vi "Control Loop.vi"(8 "error in (no error)":errorcluster, 11 "FormulaG App in":refnum<class "FormulaG App.lvclass">) -> (0 "error out":errorcluster)   [LabVIEW 2020, in "FormulaG.lvlib" / "FormulaG App.lvclass"]
uses:
  FormulaG App.lvclass
  FormulaG App.lvclass/FormulaG App.ctl
  State Update.ctl
  FormulaG-Common/Car State.ctl
  FormulaG-Common/Ranges.ctl
  FormulaG-Common/Car Info.ctl
  FormulaG-Common/Car Control.ctl
  FormulaG API/FormulaG API.lvclass
  FormulaG-Common/FormulaG-Common.lvlib
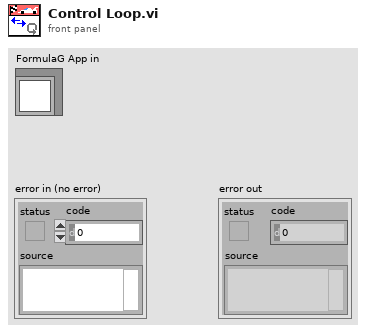
[diagram p1: front panel]
types:
  T1 = typedef "FormulaG-Common.lvlib/Control VI.ctl" = refnum<vi>
  T2 = typedef "FormulaG.lvlib/FormulaG App.lvclass/State Update.ctl" = cluster{"Car State":T3, "Car Control":T6, "Update Rate":dbl, "error":errorcluster}
  T3 = typedef "FormulaG-Common.lvlib/Car State.ctl" = cluster{"Ranges":T4, "Car Info":T5, "Current Lap":dbl, "Last Lap":dbl, "Lap":u8}
  T4 = typedef "FormulaG-Common.lvlib/Ranges.ctl" = cluster{"Front":sgl[], "Rear":sgl[]}
  T5 = typedef "FormulaG-Common.lvlib/Car Info.ctl" = cluster{"Speed":sgl, "X":sgl, "Y":sgl, "Heading":sgl}
  T6 = typedef "FormulaG-Common.lvlib/Car Control.ctl" = cluster{"Steering (-1 to 1)":sgl, "Throttle (0 to 1)":sgl}
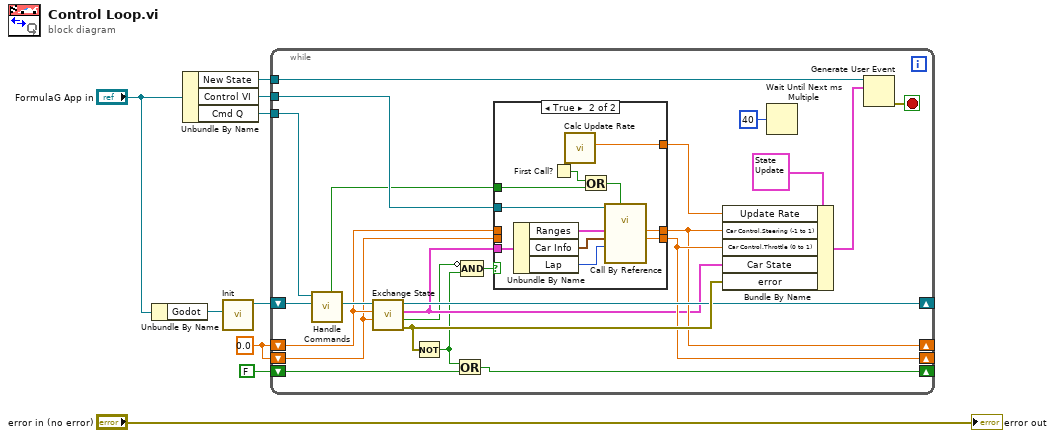
[diagram p0: block diagram]
diagram:
  w3 = sgl 0.0 ("Throttle (0 to 1)")
  n1 = Unbundle By Name("FormulaG App in") -> ("Godot"=w8:refnum<class "GodotServer.lvclass">)
  n2 = Unbundle By Name("FormulaG App in") -> ("New State"=w5:refnum<user-event>, "Control VI"=w6:T1, "Cmd Q"=w4:refnum<queue>)
  n3 = call "Init.vi"("Godot"=w8) -> ("FormulaG API out"=w2:refnum<class "FormulaG API.lvclass">)  [unwired: 9 in, 1 out]
  n4 = while {
    shift-right: [w28] -> _
    shift-left: w2 -> [w30]
    tunnel: w6 -> [w29]
    tunnel: w5 -> [w27]
    tunnel: w4 -> [w22]
    shift-right: [w20] -> _
    shift-left: w3 -> [w14]
    shift-right: [w19] -> _
    shift-left: w3 -> [w15]
    shift-right: [w16] -> _
    shift-left: FALSE -> [w18]
    stop <- w25 stop-if-true
    n5 = call "Handle Commands.vi"("FormulaG API in"=w30, "Cmd Q"=w22) -> ("FormulaG API"=w23:refnum<class "FormulaG API.lvclass">, "Reset"=w21:bool)  [unwired: 8 in]
    n6 = call "Exchange State.vi"("Throttle"=w14, "Steering"=w15, "FormulaG API in"=w23) -> ("error out"=w32:errorcluster, "Paused"=w10:bool, "Car State"=w17:T3, "FormulaG API out"=w28:refnum<class "FormulaG API.lvclass">)  [unwired: 5 in]
    n7 = Not(x=w32) -> (.not. x?=w12:bool)
    n8 = Or(x=w12, y=w18) -> (x .or. y?=w16:bool)
    n9 = Compound Arithmetic op=AND(invert w10, w12) -> (w11:bool)
    n10 = case shown="True" w11 {
      tunnel: w29 -> [_ w45]
      tunnel: w21 -> [_ w40]
      tunnel: [w33 w38] -> w20
      tunnel: [w34 w37] -> w19
      tunnel: w17 -> [_ w36]
      tunnel: w15 -> [w34 _]
      tunnel: w14 -> [w33 _]
      tunnel: [_ w35] -> w13
      frame False {
      }
      frame True {
        n11 = Unbundle By Name(w36) -> ("Ranges"=w44:T4, "Car Info"=w43:T5, "Lap"=w39:u8)
        n12 = First Call?() -> (First Call?: T/F=w42:bool)
        n13 = call "Calc Update Rate.vi"() -> ("Update Rate"=w35:dbl)  [unwired: 11 in]
        n14 = Or(x=w42, y=w40) -> (x .or. y?=w41:bool)
        n15 = call-by-ref "?"(reference=w45, "Reset"=w41, "Lap"=w39, "Car Info"=w43, "Ranges"=w44) -> ("Throttle (0 to 1)"=w38:sgl, "Steering (-1 to 1)"=w37:sgl)  [unwired: 7 in, 2 out]
      }
    }
    n16 = Bundle By Name(cluster=T2 {"Car State"={"Ranges"={"Front"=[], "Rear"=[]}, "Car Info"={"Speed"=0.0, "X"=0.0, "Y"=0.0, "Heading"=0.0}, "Current Lap"=0.0, "Last Lap"=0.0, "Lap"=0}, "Car Control"={"Steering (-1 to 1)"=0.0, "Throttle (0 to 1)"=0.0}, "Update Rate"=0.0, "error"={"status"=FALSE, "code"=0, "source"=""}} ("State Update"), "Update Rate"=w13, "Car Control.Steering (-1 to 1)"=w19, "Car Control.Throttle (0 to 1)"=w20, "Car State"=w17, "error"=w32) -> (w26:T2)
    n17 = Wait Until Next ms Multiple(millisecond multiple=u32 40 ("milliseconds to wait")) -> ()  [unwired: 1 out]
    n18 = Generate User Event(user event=w27, event data cluster=w26) -> (error out=w25:errorcluster)  [unwired: 2 in, 1 out]
  }
  "error out" <- "error in (no error)"
